vi "Anything to JSON.vi"(7 "Nested? (F)":bool, 8 "error in (no error)":errorcluster, 10 "Ignore Name? (F)":bool, 11 "Anything":variant) -> (0 "error out":errorcluster, 3 "JSON":string, 5 "Type Enum":T1)   [LabVIEW 2011, in "LV JSON.lvlib"]
uses:
  LV JSON.lvlib
  <vilib>/Utility/VariantDataType/Type.ctl
  <vilib>/Utility/error.llb/whitespace.ctl
  JSON Values/EXT to JSON Value.vi
  JSON Values/CSG to JSON Value.vi
  JSON Values/CDB to JSON Value.vi
  JSON Values/CXT to JSON Value.vi
  JSON Values/Boolean to JSON Value.vi
  JSON Values/String to JSON Value.vi
  JSON Values/DBL to JSON Value.vi
  JSON Values/I32 to JSON Value.vi
  JSON Values/U32 to JSON Value.vi
  JSON Values/I64 to JSON Value.vi
  JSON Escape.vi
  <vilib>/Utility/VariantDataType/VariantType.lvlib
panel:
  in  "utf-8 text":string
  in  "text":string
  out "text out":string
  out "utf-8 text out":string
  out "Name":string
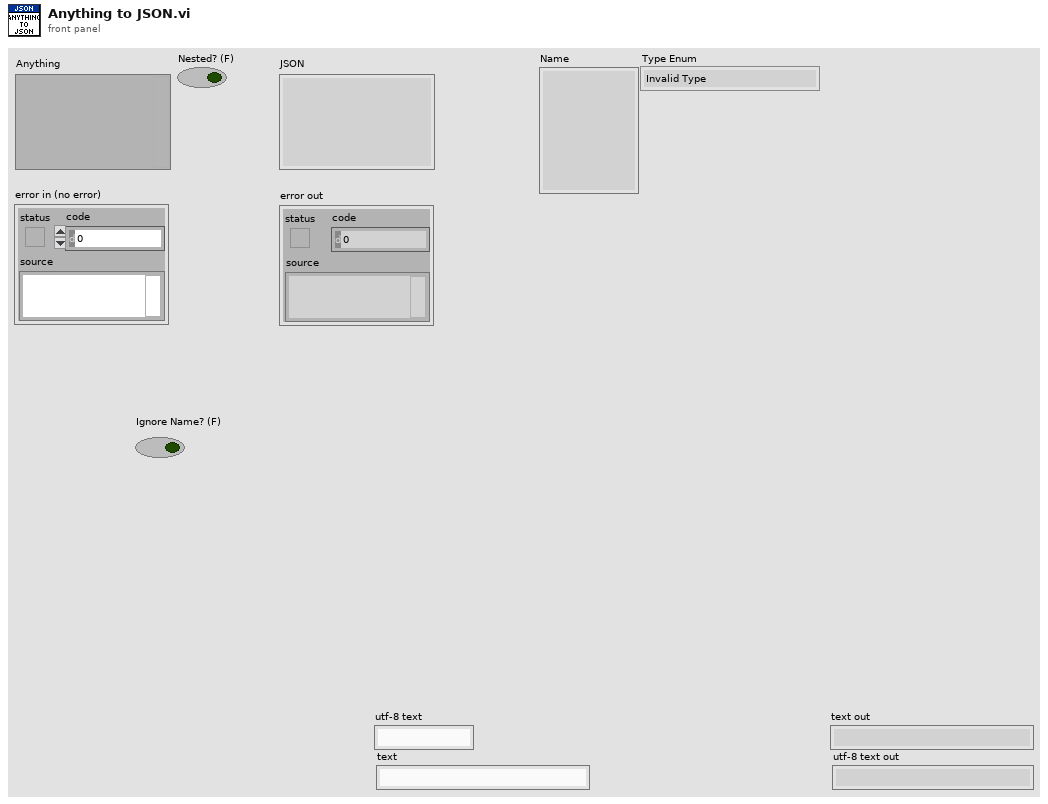
[diagram p1: front panel]
types:
  T1 = typedef "VariantType.lvlib/Type.ctl" = enum8{"Invalid Type", "Void", "I8", "I16", "I32", "I64", "U8", "U16", "U32", "U64", "Single Float", "Double Float", "Extended Float", "Single Complex", "Double Complex", "Extended Complex", "Enum U8", "Enum U16", "Enum U32", "Enum U64", "Single Float With Unit", "Double Float With Unit", "Extended Float With Unit", "Single Complex with Unit", "Double Complex with Unit", "Extended Complex with Unit", "Boolean", "String", "Path", "Picture", "Tag", "Array", "Cluster", "Variant", "LV Variant", "Waveform", "Timestamp", "Digital Waveform", "Digital Data", "ExpressData", "Refnum", "External Data", "VI", "Poly VI", "LabVIEW Class Instance", "Fixed Point"}
  T2 = typedef "imagedata.ctl" = cluster{"image type":i32, "image depth":i32, "image":u8[], "mask":u8[], "colors":u32[], "Rectangle":cluster{"left":i16, "top":i16, "right":i16, "bottom":i16}}
  T3 = typedef "whitespace.ctl" = u16
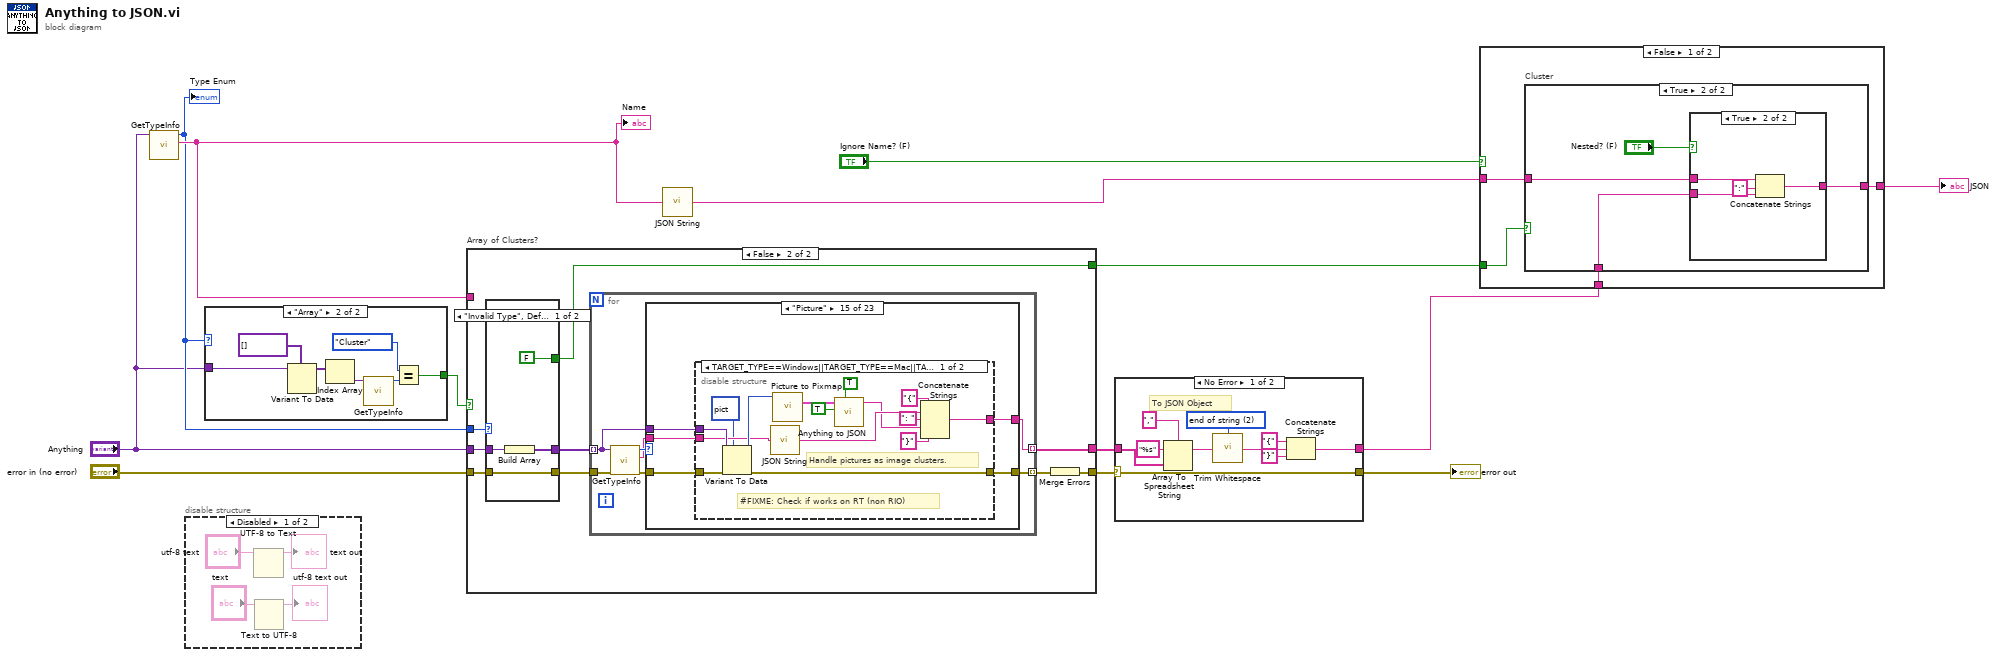
[diagram p0: block diagram]
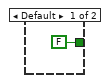
[diagram p3: hidden frame]
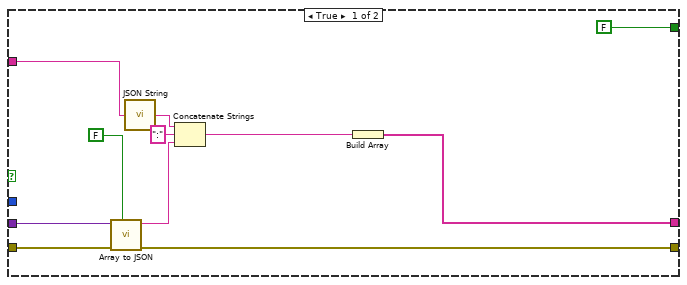
[diagram p4: hidden frame]
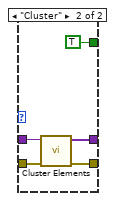
[diagram p5: hidden frame]
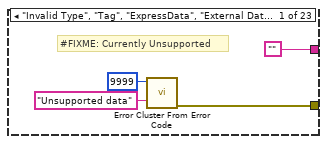
[diagram p6: hidden frame]
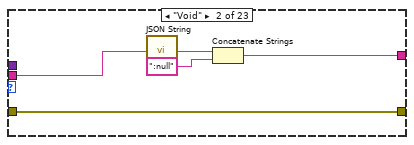
[diagram p7: hidden frame]
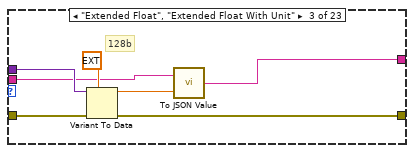
[diagram p8: hidden frame]
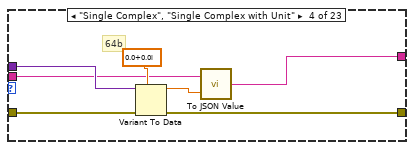
[diagram p9: hidden frame]
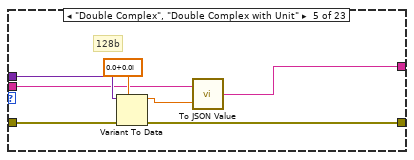
[diagram p10: hidden frame]
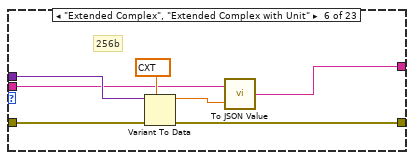
[diagram p11: hidden frame]
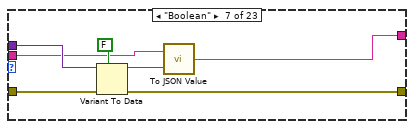
[diagram p12: hidden frame]
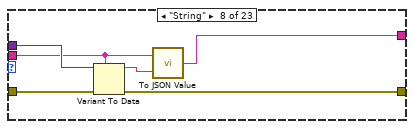
[diagram p13: hidden frame]
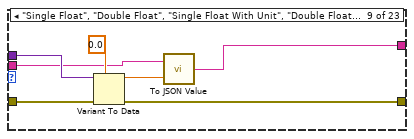
[diagram p14: hidden frame]
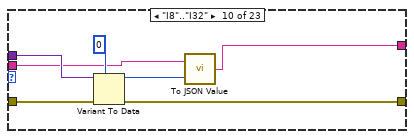
[diagram p15: hidden frame]
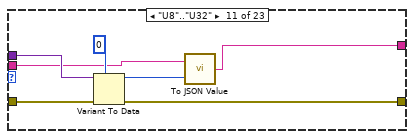
[diagram p16: hidden frame]
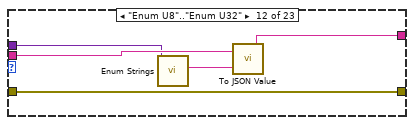
[diagram p17: hidden frame]
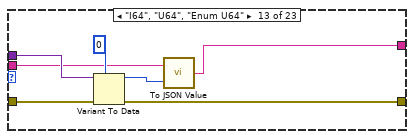
[diagram p18: hidden frame]
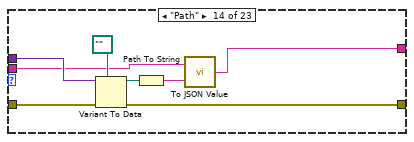
[diagram p19: hidden frame]
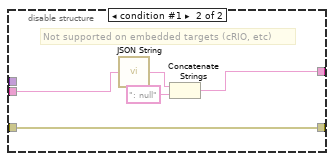
[diagram p20: hidden frame]
diagram:
  n1 = call <vilib>:"GetTypeInfo.vi"("Variant"="Anything") -> ("Name"=w5:string, "Type Enum"=w4:T1)  [unwired: 6 in, 3 out]
  "Name" <- w5
  "Type Enum" <- w4
  n2 = disable-structure shown="Disabled" {
    frame Disabled {
      n3 = UTF-8 to Text(11:"utf-8 text") -> (3:→"text out":string)  [unwired: 1 in, 1 out]
      n4 = Text to UTF-8(11:"text") -> (3:→"utf-8 text out":string)  [unwired: 1 in, 1 out]
    }
    frame Enabled {
    }
  }
  n5 = case shown="\"Array\"" w4 {
    tunnel: [FALSE w20] -> w3
    tunnel: "Anything" -> [_ w19]
    frame Default {
    }
    frame "Array" {
      n6 = Variant To Data(type=variant[] [], Variant=w19) -> (data=w23:variant[])  [unwired: 1 in, 1 out]
      n7 = Index Array(array=w23) -> (element=w24:variant)  [unwired: 1 in]
      n8 = call <vilib>:"GetTypeInfo.vi"("Variant"=w24) -> ("Type Enum"=w22:T1)  [unwired: 6 in, 4 out]
      n9 = Equal?(x=Type."Cluster" ("Type Enum"), y=w22) -> (x = y?=w20:bool)
    }
  }
  n10 = case "Array of Clusters?" shown="False" w3 {
    tunnel: "error in (no error)" -> [w31 w45]
    tunnel: [w28 w44] -> w12
    tunnel: [w30 w40] -> w8
    tunnel: w4 -> [_ w39]
    tunnel: [FALSE w38] -> w7
    tunnel: "Anything" -> [w32 w37]
    tunnel: w5 -> [w33 _]
    frame True {
      n11 = call "Array to JSON.vi"("Include Name (T)"=FALSE, "error in (no error)"=w31, "Array"=w32) -> ("error out"=w30:errorcluster, "Array in JSON"=w34:string)  [unwired: 7 in]
      n12 = call "JSON String.vi"("in"=w33) -> ("out"=w35:string)
      n13 = Concatenate Strings(w35, ":" ("string"), w34) -> (w29:string)
      n14 = Build Array(w29) -> (w28:string[])
    }
    frame False {
      n15 = case shown="\"Invalid Type\", Default" w39 {
        tunnel: w45 -> [w47 w53]
        tunnel: [w48 w51] -> w42
        tunnel: [w47 w52] -> w41
        tunnel: w37 -> [w49 w50]
        tunnel: [FALSE TRUE] -> w38
        frame "Invalid Type", Default {
          n16 = Build Array(w49) -> (w48:variant[])
        }
        frame "Cluster" {
          n17 = call "Cluster Elements.vi"("error in (no error)"=w53, "Cluster Variant"=w50) -> ("error out"=w52:errorcluster, "Cluster Elements"=w51:variant[])  [unwired: 8 in]
        }
      }
      n18 = for {
        tunnel: w42 -> [w56] mode=indexing
        tunnel: [w55] -> w44 mode=indexing
        tunnel: w41 -> [w59]
        tunnel: [w57] -> w43 mode=indexing
        n19 = call <vilib>:"GetTypeInfo.vi"("error in (no error)"=w59, "Variant"=w56) -> ("error out"=w58:errorcluster, "Name"=w60:string, "Type Enum"=w61:T1)  [unwired: 5 in, 2 out]
        n20 = case shown="\"Picture\"" w61 {
          tunnel: w56 -> [_ _ w75 w83 w89 w96 w104 w111 w118 w125 w132 w133 w144 w149 w157 w184 w191 w197 w210 w218 w228 _ w244]
          tunnel: w60 -> [_ w66 w72 w80 w87 w95 w101 w108 w114 w121 w128 w137 w139 w146 w154 w185 _ w193 w203 w214 w224 w234 w238]
          tunnel: w58 -> [_ w70 w77 w82 w90 w97 w105 w110 w117 w124 w131 w134 w143 w151 w156 w183 w188 w199 w211 w219 w229 w232 w243]
          tunnel: [w65 w70 w74 w81 w88 w93 w102 w109 w116 w123 w130 w134 w142 w150 w155 w182 w187 w196 w206 w217 w227 w232 w242] -> w57
          tunnel: ["" w67 w71 w78 w85 w92 w99 w106 w112 w119 w126 w136 w138 w145 w153 w186 w190 w194 w204 w215 w225 w233 w239] -> w55
          frame "Invalid Type", "Tag", "ExpressData", "External Data", Default {
            # "#FIXME: Currently Unsupported"
            n21 = call <vilib>:"Error Cluster From Error Code.vi"("error message (\"\")"="Unsupported data" ("error message (\"\")"), "error code (0)"=9999) -> ("error out"=w65:errorcluster)  [unwired: 7 in]
          }
          frame "Void" {
            n22 = call "JSON String.vi"("in"=w66) -> ("out"=w68:string)
            n23 = Concatenate Strings(w68, ":null" ("string")) -> (w67:string)
          }
          frame "Extended Float", "Extended Float With Unit" {
            # "128b"
            n24 = Variant To Data(error in=w77, type=ext 0.0, Variant=w75) -> (data=w73:ext, error out=w74:errorcluster)
            n25 = call-poly "To JSON Value.vi"("Value"=w73, "Name"=w72) -> ("JSON Value"=w71:string)
          }
          frame "Single Complex", "Single Complex with Unit" {
            # "64b"
            n26 = Variant To Data(error in=w82, type=csg 0.0+0.0i, Variant=w83) -> (data=w79:csg, error out=w81:errorcluster)
            n27 = call-poly "To JSON Value.vi"("Value"=w79, "Name"=w80) -> ("JSON Value"=w78:string)
          }
          frame "Double Complex", "Double Complex with Unit" {
            # "128b"
            n28 = Variant To Data(error in=w90, type=cdb 0.0+0.0i, Variant=w89) -> (data=w86:cdb, error out=w88:errorcluster)
            n29 = call-poly "To JSON Value.vi"("Value"=w86, "Name"=w87) -> ("JSON Value"=w85:string)
          }
          frame "Extended Complex", "Extended Complex with Unit" {
            # "256b"
            n30 = Variant To Data(error in=w97, type=cxt 0.0+0.0i, Variant=w96) -> (data=w94:cxt, error out=w93:errorcluster)
            n31 = call-poly "To JSON Value.vi"("Value"=w94, "Name"=w95) -> ("JSON Value"=w92:string)
          }
          frame "Boolean" {
            n32 = Variant To Data(error in=w105, type=FALSE, Variant=w104) -> (data=w100:bool, error out=w102:errorcluster)
            n33 = call-poly "To JSON Value.vi"("Value"=w100, "Name"=w101) -> ("JSON Value"=w99:string)
          }
          frame "String" {
            n34 = Variant To Data(error in=w110, type=w108, Variant=w111) -> (data=w107:string, error out=w109:errorcluster)
            n35 = call-poly "To JSON Value.vi"("Value"=w107, "Name"=w108) -> ("JSON Value"=w106:string)
          }
          frame "Single Float", "Double Float", "Single Float With Unit", "Double Float With Unit", "Fixed Point" {
            n36 = Variant To Data(error in=w117, type=0.0, Variant=w118) -> (data=w113:dbl, error out=w116:errorcluster)
            n37 = call-poly "To JSON Value.vi"("Value"=w113, "Name"=w114) -> ("JSON Value"=w112:string)
          }
          frame "I8".."I32" {
            n38 = Variant To Data(error in=w124, type=0, Variant=w125) -> (data=w120:i32, error out=w123:errorcluster)
            n39 = call-poly "To JSON Value.vi"("Value"=w120, "Name"=w121) -> ("JSON Value"=w119:string)
          }
          frame "U8".."U32" {
            n40 = Variant To Data(error in=w131, type=u32 0, Variant=w132) -> (data=w127:u32, error out=w130:errorcluster)
            n41 = call-poly "To JSON Value.vi"("Value"=w127, "Name"=w128) -> ("JSON Value"=w126:string)
          }
          frame "Enum U8".."Enum U32" {
            n42 = call "Enum Strings.vi"("Enum"=w133) -> ("Selected item"=w135:string)  [unwired: 8 in, 2 out]
            n43 = call-poly "To JSON Value.vi"("Value"=w135, "Name"=w137) -> ("JSON Value"=w136:string)
          }
          frame "I64", "U64", "Enum U64" {
            n44 = Variant To Data(error in=w143, type=i64 0, Variant=w144) -> (data=w140:i64, error out=w142:errorcluster)
            n45 = call-poly "To JSON Value.vi"("Value"=w140, "Name"=w139) -> ("JSON Value"=w138:string)
          }
          frame "Path" {
            n46 = Variant To Data(error in=w151, type=path "", Variant=w149) -> (data=w148:path, error out=w150:errorcluster)
            n47 = Path To String(path=w148) -> (string=w147:string)
            n48 = call-poly "To JSON Value.vi"("Value"=w147, "Name"=w146) -> ("JSON Value"=w145:string)
          }
          frame "Picture" {
            n49 = disable-structure shown="TARGET_TYPE==Windows||TARGET_TYPE==Mac||TARGET_TYPE==Unix" {
              disable-tunnel: w157 -> [w172 _]
              disable-tunnel: w156 -> [w171 w175]
              disable-tunnel: [w168 w175] -> w155
              disable-tunnel: w154 -> [w161 w174]
              disable-tunnel: [w159 w173] -> w153
              frame condition #0 (active) {
                # "#FIXME: Check if works on RT (non RIO)"
                # "Handle pictures as image clusters."
                n50 = Variant To Data(error in=w171, type=picture data[5B] ("empty picture"), Variant=w172) -> (data=w170:picture, error out=w168:errorcluster)
                n51 = call "JSON String.vi"("in"=w161) -> ("out"=w162:string)
                n52 = call <vilib>:"Picture to Pixmap.vi"("picture"=w170) -> ("image data"=w169:T2)  [unwired: 9 in, 1 out]
                n53 = call "Anything to JSON.vi"("Nested? (F)"=TRUE, "Ignore Name? (F)"=TRUE, "Anything"=w169) -> ("JSON"=w160:string)  [unwired: 6 in, 2 out]
                n54 = Concatenate Strings("{", w162, ": " ("string"), w160, "}") -> (w159:string)
              }
              frame condition #1 {
                # "Not supported on embedded targets (cRIO, etc)"
                n55 = call "JSON String.vi"("in"=w174) -> ("out"=w176:string)
                n56 = Concatenate Strings(w176, ": null" ("string")) -> (w173:string)
              }
            }
          }
          frame "Array" {
            n57 = call "Array to JSON.vi"("Include Name (T)"=FALSE, "error in (no error)"=w183, "Array"=w184) -> ("error out"=w182:errorcluster, "Array in JSON"=w179:string)  [unwired: 7 in]
            n58 = call "JSON String.vi"("in"=w185) -> ("out"=w180:string)
            n59 = Concatenate Strings(w180, ":" ("string"), w179) -> (w186:string)
          }
          frame "Cluster" {
            n60 = call "Anything to JSON.vi"("Nested? (F)"=TRUE, "error in (no error)"=w188, "Anything"=w191) -> ("error out"=w187:errorcluster, "JSON"=w190:string)  [unwired: 6 in, 1 out]
          }
          frame "Variant", "LV Variant", "VI".."LabVIEW Class Instance" {
            # "#FIXME: Currently Unsupported"
            n61 = Variant To Data(error in=w199, type=variant ("variant"), Variant=w197) -> (data=w201:variant, error out=w200:errorcluster)
            n62 = Flatten To String(anything=w201, error in (no error)=w200) -> (error out=w196:errorcluster)  [unwired: 2 in, 2 out]
            n63 = call "JSON String.vi"("in"=w193) -> ("out"=w192:string)
            n64 = Concatenate Strings(w192, ": null" ("string")) -> (w194:string)
          }
          frame "Waveform" {
            # "#FIXME: Currently Unsupported"
            n65 = Variant To Data(error in=w211, type=waveform(dbl) {"t0"=timestamp(0 s since 1904-01-01), "dt"=1.0, "Y"=[]} ("waveform"), Variant=w210) -> (data=w208:waveform(dbl), error out=w207:errorcluster)
            n66 = Flatten To String(anything=w208, error in (no error)=w207) -> (error out=w206:errorcluster)  [unwired: 2 in, 2 out]
            n67 = call "JSON String.vi"("in"=w203) -> ("out"=w202:string)
            n68 = Concatenate Strings(w202, ": null" ("string")) -> (w204:string)
          }
          frame "Digital Waveform" {
            # "#FIXME: Currently Unsupported"
            n69 = Variant To Data(error in=w219, type=digitalwaveform {"t0"=timestamp(0 s since 1904-01-01), "dt"=0.0, "Y"={"transitions"=[], "data"=[]}, "error"={"status"=FALSE, "code"=37421928, "source"=""}} ("digital waveform out"), Variant=w218) -> (data=w221:digitalwaveform, error out=w220:errorcluster)
            n70 = Flatten To String(anything=w221, error in (no error)=w220) -> (error out=w217:errorcluster)  [unwired: 2 in, 2 out]
            n71 = call "JSON String.vi"("in"=w214) -> ("out"=w213:string)
            n72 = Concatenate Strings(w213, ": null" ("string")) -> (w215:string)
          }
          frame "Digital Data" {
            # "#FIXME: Currently Unsupported"
            n73 = Variant To Data(error in=w229, type=digitaldata {"transitions"=[], "data"=[]} ("digital data"), Variant=w228) -> (data=w231:digitaldata, error out=w230:errorcluster)
            n74 = Flatten To String(anything=w231, error in (no error)=w230) -> (error out=w227:errorcluster)  [unwired: 2 in, 2 out]
            n75 = call "JSON String.vi"("in"=w224) -> ("out"=w223:string)
            n76 = Concatenate Strings(w223, ": null" ("string")) -> (w225:string)
          }
          frame "Refnum" {
            # "#FIXME: Currently Unsupported"
            n77 = call "JSON String.vi"("in"=w234) -> ("out"=w235:string)
            n78 = Concatenate Strings(w235, ": null" ("string")) -> (w233:string)
          }
          frame "Timestamp" {
            n79 = Variant To Data(error in=w243, type=timestamp(0 s since 1904-01-01) ("refnum"), Variant=w244) -> (data=w241:timestamp, error out=w242:errorcluster)
            n80 = Format Date/Time String(time format string (%c)="%02m/%02d/%Y %H:%M:%S%03u", seconds (now)=w241) -> (date/time string=w237:string)  [unwired: 1 in]
            n81 = call-poly "To JSON Value.vi"("Value"=w237, "Name"=w238) -> ("JSON Value"=w239:string)
          }
        }
      }
      n82 = Merge Errors(w43) -> (w40:errorcluster)
    }
  }
  n83 = call "JSON String.vi"("in"=w5) -> ("out"=w10:string)
  n84 = case shown="No Error" w8 {
    selector: w8 -> [w255 w256]
    tunnel: [w255 w256] -> w11
    tunnel: w12 -> [w253 _]
    tunnel: [w250 _] -> w9
    frame No Error {
      w246 = T3 2 items=["both", "start of string", "end of string"] ("location (both)")
      # "To JSON Object"
      n85 = Array To Spreadsheet String(delimiter (Tab)=",", array=w253, 3:"%s" ("delimiter (Tab)")) -> (spreadsheet string=w254:string)
      n86 = call <vilib>:"Trim Whitespace.vi"("string"=w254, "location (both)"=w246) -> ("trimmed string"=w247:string)
      n87 = Concatenate Strings("{" ("string"), w247, "}" ("string")) -> (w250:string)
    }
    frame Error {
    }
  }
  "error out" <- w11
  n88 = case shown="False" "Ignore Name? (F)" {
    tunnel: w10 -> [w260 _]
    tunnel: [w259 w276] -> w1
    tunnel: w9 -> [w258 w276]
    tunnel: w7 -> [w257 _]
    frame False {
      n89 = case "Cluster" shown="True" w257 {
        tunnel: w260 -> [_ w265]
        tunnel: [w261 w264] -> w259
        tunnel: w258 -> [w261 w263]
        frame False {
        }
        frame True {
          n90 = case shown="True" "Nested? (F)" {
            tunnel: w265 -> [w271 w275]
            tunnel: [w270 w274] -> w264
            tunnel: w263 -> [w269 w273]
            frame False {
              n91 = Concatenate Strings("{" ("string"), w271, ":" ("string"), w269, "}" ("string")) -> (w270:string)
            }
            frame True {
              n92 = Concatenate Strings(w275, ":" ("string"), w273) -> (w274:string)
            }
          }
        }
      }
    }
    frame True {
    }
  }
  "JSON" <- w1
